vi "Check Database For Entry Errors.vi"(7 "All Parameters Array":T1[](array[typedef])) -> (8 "Database OK?":bool)   [LabVIEW 2020]
uses:
  Controls/Database_Array.ctl
  Controls/Encoding.ctl
  Get Active List - By Core Number.vi
  Parameter Filter - By Core Number.vi
  Get Active List - By Channel Number.vi
  Parameter Filter - By Channel Number.vi
  Get Active List - By Label Decimal.vi
  Parameter Filter - By Label Decimal.vi
  Get Active List - By SDI.vi
  Parameter Filter - By SDI.vi
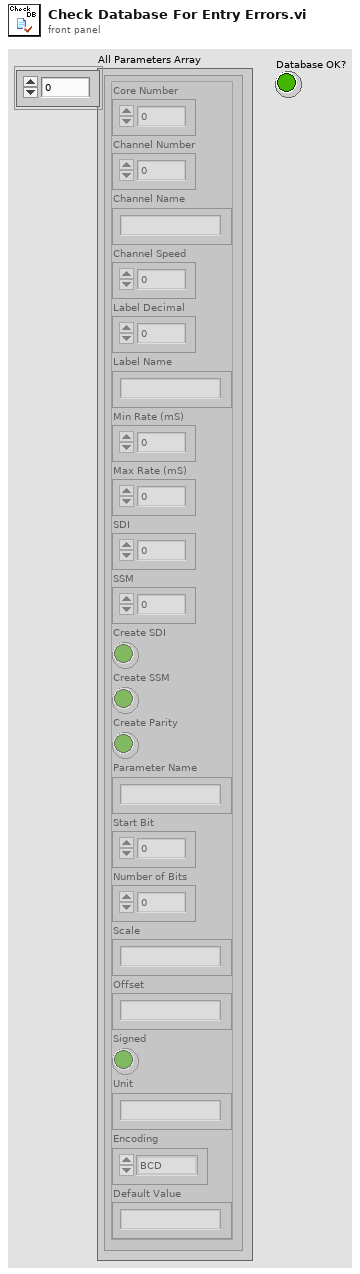
[diagram p1: front panel]
types:
  T1 = typedef "Database_Array.ctl" = cluster{"Core Number":i32, "Channel Number":i32, "Channel Name":string, "Channel Speed":i32, "Label Decimal":i32, "Label Name":string, "Min Rate (mS)":i32, "Max Rate (mS)":i32, "SDI":i32, "SSM":i32, "Create SDI":bool, "Create SSM":bool, "Create Parity":bool, "Parameter Name":string, "Start Bit":i32, "Number of Bits":i32, "Scale":string, "Offset":string, "Signed":bool, "Unit":string, "Encoding":T2, "Default Value":string}
  T2 = typedef "Encoding.ctl" = enum16{"BCD", "BNR", "Discrete"}
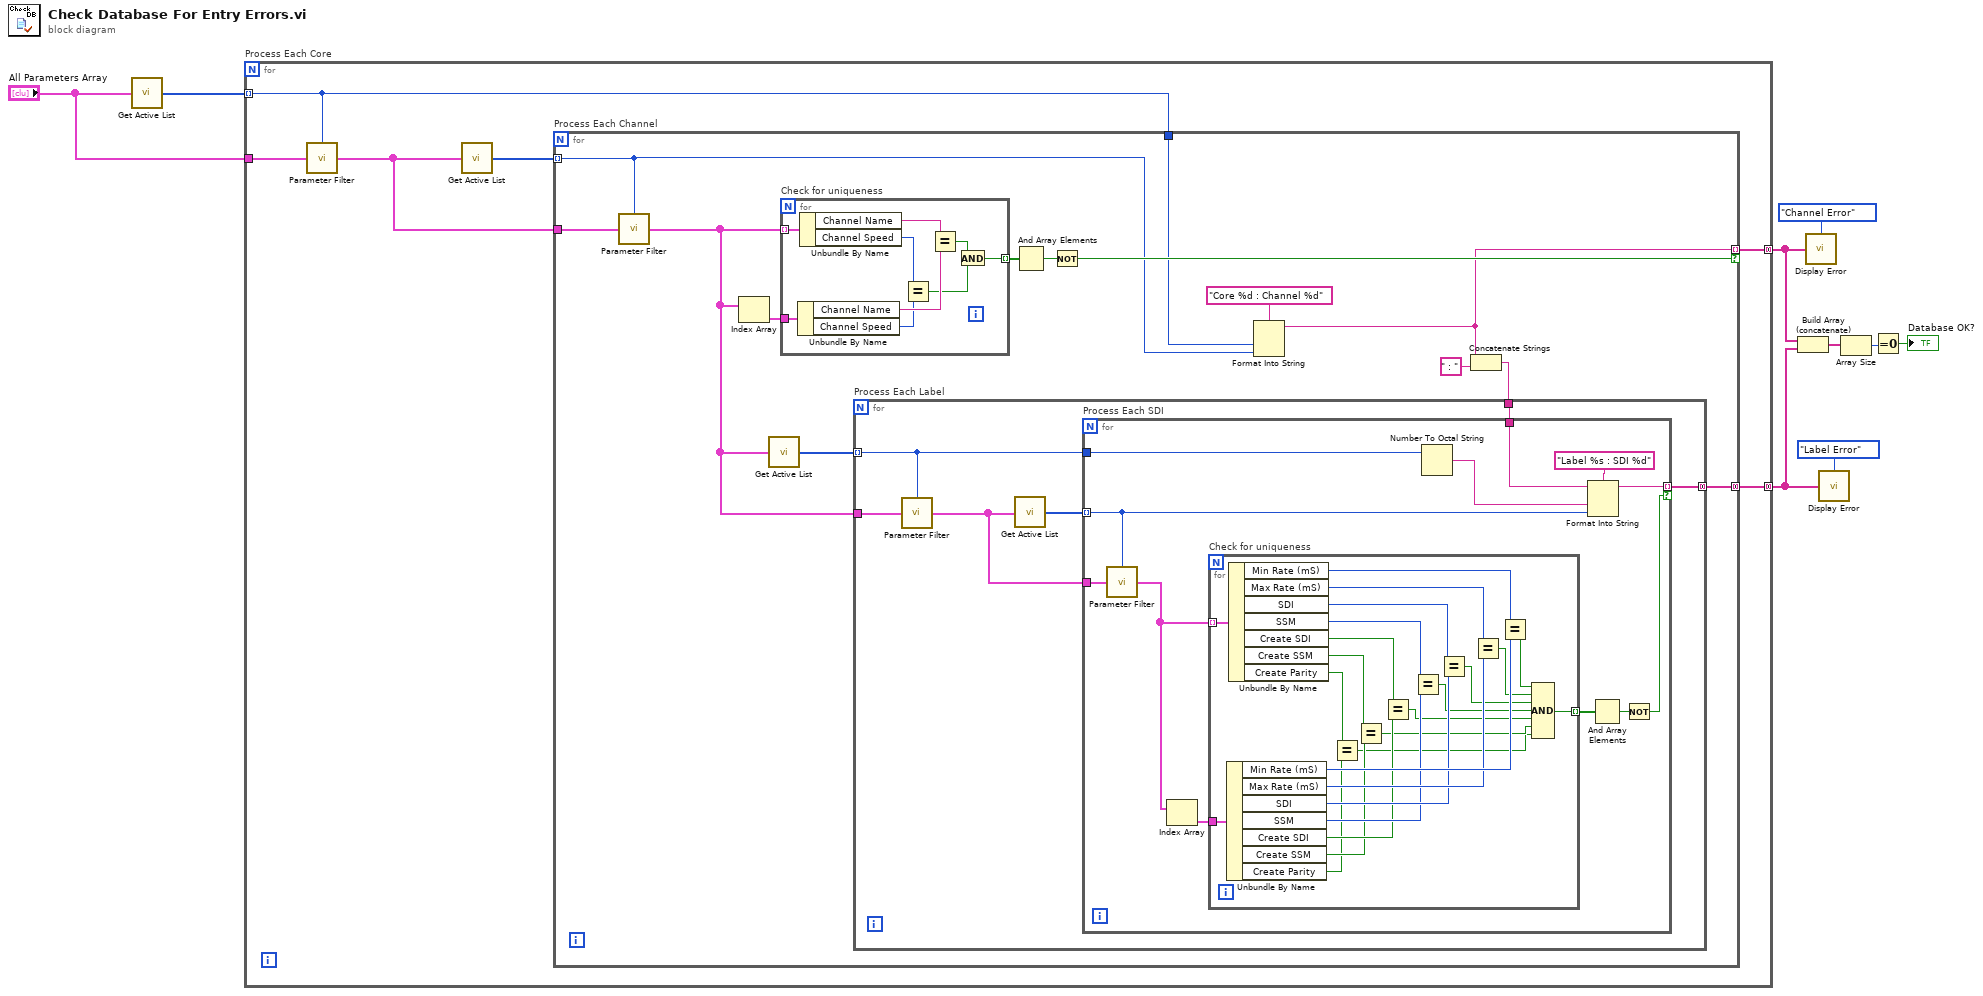
[diagram p0: block diagram]
diagram:
  n1 = call-poly "Get Active List.vi"("Parameters Array (in)"="All Parameters Array") -> ("Active Core Numbers"=w9:i32[])  [unwired: 14 in]
  n2 = for "Process Each Core" {
    tunnel: w9 -> [w10] mode=indexing
    tunnel: "All Parameters Array" -> [w15]
    tunnel: [w12] -> w5 mode=concatenating
    tunnel: [w11] -> w4 mode=concatenating
    n3 = call-poly "Parameter Filter.vi"("Core Number"=w10, "Parameters Array (in)"=w15) -> ("Filtered Parameters Array (out)"=w13:T1[])  [unwired: 13 in]
    n4 = call-poly "Get Active List.vi"("Parameters Array (in)"=w13) -> ("Active Channel Numbers"=w14:i32[])  [unwired: 14 in]
    n5 = for "Process Each Channel" {
      tunnel: w14 -> [w19] mode=indexing
      tunnel: w13 -> [w29]
      tunnel: [w18] -> w12 mode=indexing if=w25
      tunnel: [w22] -> w11 mode=concatenating
      tunnel: w10 -> [w20]
      n6 = call-poly "Parameter Filter.vi"("Channel Number"=w19, "Parameters Array (in)"=w29) -> ("Filtered Parameters Array (out)"=w23:T1[])  [unwired: 13 in]
      n7 = Index Array(array=w23) -> (element=w26:T1)  [unwired: 1 in]
      n8 = call-poly "Get Active List.vi"("Parameters Array (in)"=w23) -> ("Active Label Decimals"=w24:i32[])  [unwired: 14 in]
      n9 = for "Check for uniqueness" {
        tunnel: w23 -> [w80] mode=indexing
        tunnel: w26 -> [w79]
        tunnel: [w72] -> w27 mode=indexing
        n10 = Unbundle By Name(w79) -> ("Channel Name"=w77:string, "Channel Speed"=w76:i32)
        n11 = Unbundle By Name(w80) -> ("Channel Name"=w78:string, "Channel Speed"=w75:i32)
        n12 = Equal?(x=w75, y=w76) -> (x = y?=w73:bool)
        n13 = Equal?(x=w78, y=w77) -> (x = y?=w74:bool)
        n14 = And(x=w74, y=w73) -> (x .and. y?=w72:bool)
      }
      n15 = And Array Elements(Boolean array=w27) -> (logical AND=w28:bool)
      n16 = Not(x=w28) -> (.not. x?=w25:bool)
      n17 = Format Into String(format string="Core %d : Channel %d", w20, w19) -> (resulting string=w18:string)  [unwired: 2 in, 1 out]
      n18 = Concatenate Strings(w18, " : " ("string")) -> (w16:string)
      n19 = for "Process Each Label" {
        tunnel: w24 -> [w30] mode=indexing
        tunnel: w23 -> [w35]
        tunnel: [w32] -> w22 mode=concatenating
        tunnel: w16 -> [w31]
        n20 = call-poly "Parameter Filter.vi"("Label Decimal"=w30, "Parameters Array (in)"=w35) -> ("Filtered Parameters Array (out)"=w33:T1[])  [unwired: 13 in]
        n21 = call-poly "Get Active List.vi"("Parameters Array (in)"=w33) -> ("Active SDIs"=w34:i32[])  [unwired: 14 in]
        n22 = for "Process Each SDI" {
          tunnel: w34 -> [w40] mode=indexing
          tunnel: w33 -> [w47]
          tunnel: [w38] -> w32 mode=indexing if=w42
          tunnel: w31 -> [w39]
          tunnel: w30 -> [w37]
          n23 = call-poly "Parameter Filter.vi"("SDI"=w40, "Parameters Array (in)"=w47) -> ("Filtered Parameters Array (out)"=w45:T1[])  [unwired: 13 in]
          n24 = Index Array(array=w45) -> (element=w44:T1)  [unwired: 1 in]
          n25 = for "Check for uniqueness" {
            tunnel: w45 -> [w71] mode=indexing
            tunnel: [w48] -> w43 mode=indexing
            tunnel: w44 -> [w66]
            n26 = Unbundle By Name(w66) -> ("Min Rate (mS)"=w69:i32, "Max Rate (mS)"=w68:i32, "SDI"=w64:i32, "SSM"=w62:i32, "Create SDI"=w60:bool, "Create SSM"=w58:bool, "Create Parity"=w56:bool)
            n27 = Unbundle By Name(w71) -> ("Min Rate (mS)"=w70:i32, "Max Rate (mS)"=w67:i32, "SDI"=w65:i32, "SSM"=w63:i32, "Create SDI"=w61:bool, "Create SSM"=w59:bool, "Create Parity"=w57:bool)
            n28 = Equal?(x=w57, y=w56) -> (x = y?=w49:bool)
            n29 = Equal?(x=w59, y=w58) -> (x = y?=w50:bool)
            n30 = Equal?(x=w61, y=w60) -> (x = y?=w51:bool)
            n31 = Equal?(x=w63, y=w62) -> (x = y?=w52:bool)
            n32 = Equal?(x=w65, y=w64) -> (x = y?=w53:bool)
            n33 = Equal?(x=w67, y=w68) -> (x = y?=w54:bool)
            n34 = Equal?(x=w70, y=w69) -> (x = y?=w55:bool)
            n35 = Compound Arithmetic op=AND(w55, w54, w53, w52, w51, w50, w49) -> (w48:bool)
          }
          n36 = Number To Octal String(2:w37) -> (0:w36:string)  [unwired: 1 in]
          n37 = Format Into String(format string="Label %s : SDI %d", initial string=w39, w36, w40) -> (resulting string=w38:string)  [unwired: 1 in, 1 out]
          n38 = And Array Elements(Boolean array=w43) -> (logical AND=w46:bool)
          n39 = Not(x=w46) -> (.not. x?=w42:bool)
        }
      }
    }
  }
  n40 = Build Array (concatenate)(w5, w4) -> (w3:string[])
  n41 = call "Display Error.vi"("Error Type"=enum16{"Channel Error", "Label Error"}."Channel Error", "Errors"=w5) -> ()  [unwired: 14 in]
  n42 = call "Display Error.vi"("Error Type"=enum16{"Channel Error", "Label Error"}."Label Error", "Errors"=w4) -> ()  [unwired: 14 in]
  n43 = Array Size(array=w3) -> (size(s)=w2:i32)
  n44 = Equal To 0?(x=w2) -> (x = 0?=→"Database OK?":bool)
